vi "FinalizeTurn.vi"(6 "Error":errorcluster, 7 "Actor":refnum<class "Actor Layer.lvclass">) -> (4 "Error":errorcluster, 5 "Actor":refnum<class "Actor Layer.lvclass">)   [LabVIEW 2020, in "_Template.lvlib" / "{{Actor}}.lvlib" / "Actor Layer.lvclass"]
uses:
  Actor Layer.lvclass
  Actor Layer.lvclass/Actor Layer.ctl
  jettl/jettl/Actor Layer/Actor Layer.lvclass
panel:
  # "This front panel should not be manipulated."
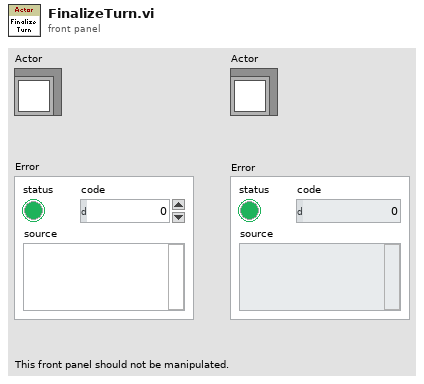
[diagram p1: front panel]
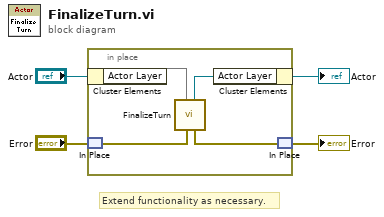
[diagram p0: block diagram]
diagram:
  # "Extend functionality as necessary."
  n1 = in-place {
    n2 = in-place-cluster #1("Actor") -> ("Actor Layer"=w8)
    n3 = in-place-match #2("Error") -> (w6:errorcluster)
    n4 = call-dynamic "FinalizeTurn.vi"("Error"=w6, "Actor"=w8) -> ("Error"=w5:errorcluster, "Actor"=w7:refnum<class "Actor Layer.lvclass">)  [unwired: 7 in, 1 out]
    n5 = in-place-cluster #1("Actor Layer"=w7) -> (→"Actor":refnum<class "Actor Layer.lvclass">)
    n6 = in-place-match #2(w5) -> (→"Error":errorcluster)
  }
